vi "ArrayFindClosestValue.vi"(10 "Search Item":dbl, 11 "Array":dbl[](array[numeric])) -> (3 "Index":i32)   [LabVIEW 2021]
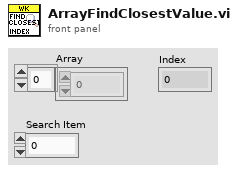
[diagram p1: front panel]
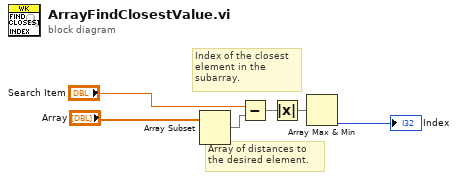
[diagram p0: block diagram]
diagram:
  # "Index of the closest element in the subarray."
  # "Array of distances to the desired element."
  n1 = Array Subset(array="Array") -> (w3:dbl[])  [unwired: 2 in]
  n2 = Subtract(x="Search Item", y=w3) -> (x-y=w1:dbl[])
  n3 = Absolute Value(x=w1) -> (abs(x)=w2:dbl[])
  n4 = Array Max & Min(array=w2) -> (min index (indices)=→"Index":i32)  [unwired: 3 out]
